vi "JK_FlipFlop.vi"(2 "K":bool, 3 "CLK":bool, 4 "J":bool) -> (0 "__\nQ":bool, 1 "Q":bool)   [LabVIEW 2018]
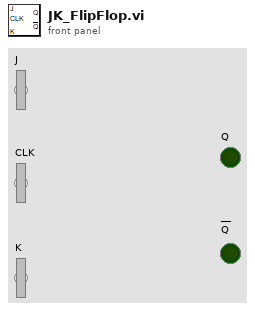
[diagram p1: front panel]
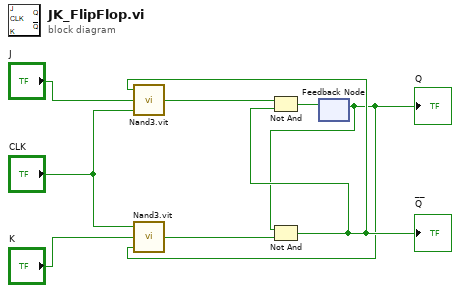
[diagram p0: block diagram]
diagram:
  n1 = feedback #1() -> (w1:bool)  [unwired: 1 in]
  "Q" <- w1
  n2 = call "Nand3.vit"("C"=w1, "B"="K", "A"="CLK") -> ("Boolean"=w7:bool)
  n3 = Not And(1:w7, 2:w1) -> (0:w2:bool)
  "__\nQ" <- w2
  n4 = call "Nand3.vit"("C"="CLK", "B"="J", "A"=w2) -> ("Boolean"=w6:bool)
  n5 = Not And(1:w2, 2:w6) -> (0:w8:bool)
  n6 = feedback-in #1(w8) -> ()
